vi "Extract data from spreadsheet (subVi).vi"(0 "file path (dialog if empty)":path, 1 "error in (no error)":errorcluster) -> (2 "new file path (Not A Path if cancelled)":path, 3 "data out":dbl[][](array[numeric]), 4 "error out":errorcluster)   [LabVIEW 2016]
uses:
  <vilib>/Utility/file.llb/Read Delimited Spreadsheet (string).vi
panel:
  out "time":string
  out "mass":dbl
  out "pressure":dbl
  out "date":string
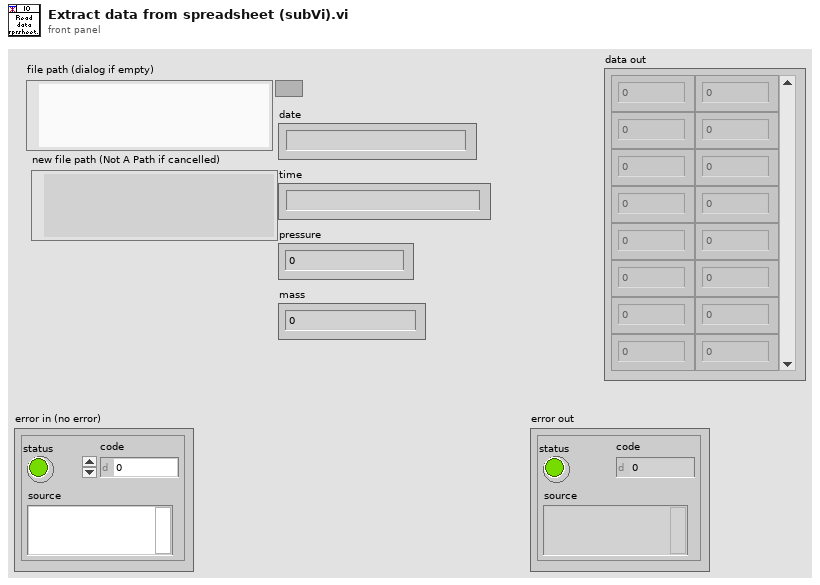
[diagram p1: front panel]
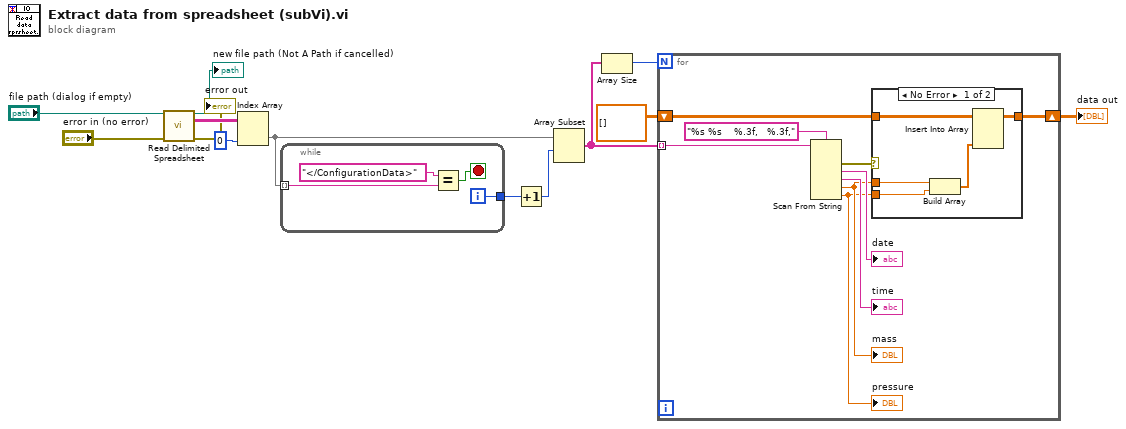
[diagram p0: block diagram]
diagram:
  n1 = call-poly <vilib>:"Read Delimited Spreadsheet.vi"("file path (dialog if empty)"="file path (dialog if empty)", "error in (no error)"="error in (no error)") -> ("new file path (Not A Path if cancelled)"=→"new file path (Not A Path if cancelled)":path, "all rows"=w13:string[][], "error out"=→"error out":errorcluster)  [unwired: 8 in, 3 out]
  n2 = Index Array(array=w13, index (col)=0 ("disabled index (col)")) -> (element=w11:string[])  [unwired: 1 in]
  n3 = while {
    tunnel: w11 -> [w17] mode=indexing
    tunnel: [w14] -> w10
    i -> [w14]
    stop <- w15 stop-if-true
    n4 = Equal?(x="</ConfigurationData>", y=w17) -> (x = y?=w15:bool)
  }
  n5 = Increment(x=w10) -> (x+1=w9:i32)
  n6 = Array Subset(array=w11, index=w9) -> (w6:string[])  [unwired: 1 in]
  n7 = Array Size(array=w6) -> (size(s)=w7:i32)
  n8 = for {
    N: w7 -> [_]
    tunnel: w6 -> [w23] mode=indexing
    shift-right: [w19] -> w4
    shift-left: dbl[][] [] -> [w20]
    n9 = Scan From String(format string="%s %s    %.3f,   %.3f,", input string=w23) -> (error out=w18:errorcluster, output 1=→"date":string, output 2=→"time":string, output 3=w22:dbl, output 4=w21:dbl)  [unwired: 6 in, 2 out]
    "pressure" <- w21
    "mass" <- w22
    n10 = case shown="No Error" w18 {
      tunnel: w22 -> [w31 _]
      tunnel: w21 -> [w30 _]
      tunnel: w20 -> [w29 w32]
      tunnel: [w27 w32] -> w19
      frame No Error {
        n11 = Build Array(w31, w30) -> (w28:dbl[])
        n12 = Insert Into Array(array=w29, new element=w28) -> (w27:dbl[][])  [unwired: 2 in]
      }
      frame Error {
      }
    }
  }
  "data out" <- w4
